vi "Shoot.vi"(5 "Joystick":dbl, 6 "Aimbot?":bool=TRUE, 7 "Aimbot Transformations":T1={"AngleThreshold(degrees)"=100.0, "ShotDuration(10ms)"=100, "PowerScale"=1.0, "AngleShift"=0}, 8 "error in":errorcluster, 9 "Spinup Trigger":bool, 10 "Trigger":bool, 11 "Vision Distance":dbl) -> (0 "error out":errorcluster, 2 "LaunchSpeed(RPM)":dbl, 3 "AngleMotorPosition(Position or %Volts)":dbl)   [LabVIEW 2015]
doc: "Collects and fires boulders according to the following parameters:\n\nTrigger: True will fire the boulder.\nSpinup Trigger: True will spin wheels up prior to firing.\nCollection Trigger: True will spin wheels backwards to collect a boulder.\nAimbot Transformations: Corrective inputs used if we are consistently over/under shooting.\nManual Control: If vision doesn't work, then aim manually using these joystick inputs."
uses:
  Robot Global Data.vi
panel:
  in  "Shot Speed Control":dbl
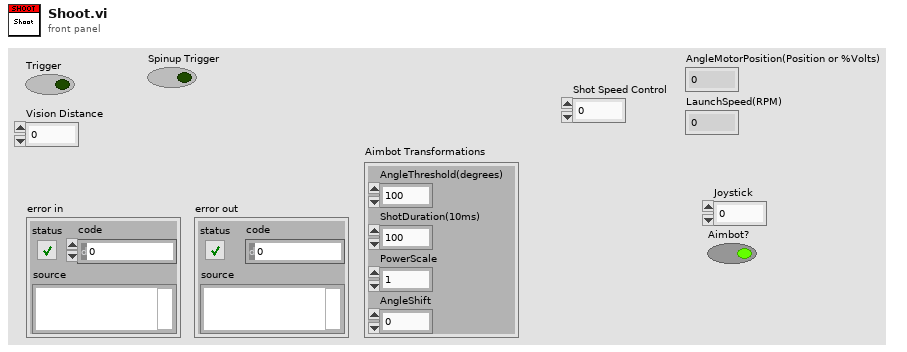
[diagram p1: front panel]
types:
  T1 = cluster{"AngleThreshold(degrees)":dbl, "ShotDuration(10ms)":i32, "PowerScale":dbl, "AngleShift":i32}
  T2 = typedef "Bundle.ctl" = cluster{"error":errorcluster, "AngleMotorRefnum":T3, "LeftWheelRefnum":T3, "RightWheelRefnum":T3, "PushSolenoidRefnum":T10, "AngleMotorPosition(Position or %Volts)":dbl, "LaunchSpeed(RPM)":dbl, "CollectSpeed(RPM)":dbl, "AngleThreshold":dbl, "ShotDuration(10ms)":i32}
  T3 = typedef "WPI_MotorControlDeviceRef.ctl" = cluster{"DeviceStatus":errorcluster, "Type":T4, "PWM":cluster{"PWM Channel":T5, "DeadBand":T6}, "CAN":cluster{"Device Number":u8, "Control Mode":T7, "Semaphore":T8, "Max Vout":dbl, "TalonSRX Control Mode":T9}, "Invert":bool}
  T4 = typedef "WPI_MotorControlType.ctl" = enum16{"PWM", "CAN", "CANTalonSRX"}
  T5 = typedef "FPGA_DIOPWMChannel.ctl" = enum8{"PWM 0", "PWM 1", "PWM 2", "PWM 3", "PWM 4", "PWM 5", "PWM 6", "PWM 7", "PWM 8", "PWM 9", "PWM MXP 0", "PWM MXP 1", "PWM MXP 2", "PWM MXP 3", "PWM MXP 4", "PWM MXP 5", "PWM MXP 6", "PWM MXP 7", "PWM MXP 8", "PWM MXP 9", "Invalid"}
  T6 = typedef "WPI_PWMDeadband.ctl" = cluster{"Name":string, "maxPositivePwm":i32, "minPositivePwm":i32, "centerPwm":i32, "maxNegativePwm":i32, "minNegativePwm":i32, "angularRange":u16}
  T7 = typedef "WPI_CANJaguar_ControlMode.ctl" = enum8{"Percent VBus", "Current", "Speed", "Position", "Voltage"}
  T8 = typedef "Semaphore RefNum" = refnum<k1>
  T9 = typedef "WPI_CANTalonSRX_APIControlMode.ctl" = enum8{"Percent VBus", "Speed", "Position", "Slave", "Unchanged / Invalid", "Voltage Compensation", "Current", "Motion Profile"}
  T10 = typedef "WPI_SolenoidDevRef.ctl" = cluster{"DevStatus":errorcluster, "Pneumatics Control Module":u8, "Forward Solenoid Channel":T11, "Reverse Solenoid Channel":T11}
  T11 = typedef "WPI_SolenoidChannel.ctl" = enum8{"Solenoid 0", "Solenoid 1", "Solenoid 2", "Solenoid 3", "Solenoid 4", "Solenoid 5", "Solenoid 6", "Solenoid 7", "Invalid"}
  T12 = typedef "WPI_DigitalInputDevRef.ctl" = cluster{"DevStatus":errorcluster, "DIO Channel":T13}
  T13 = typedef "FPGA_DIOChannel.ctl" = enum8{"DIO 0", "DIO 1", "DIO 2", "DIO 3", "DIO 4", "DIO 5", "DIO 6", "DIO 7", "DIO 8", "DIO 9", "DIO MXP 0", "DIO MXP 1", "DIO MXP 2", "DIO MXP 3", "DIO MXP 4", "DIO MXP 5", "DIO MXP 6", "DIO MXP 7", "DIO MXP 8", "DIO MXP 9", "DIO MXP 10", "DIO MXP 11", "DIO MXP 12", "DIO MXP 13", "DIO MXP 14", "DIO MXP 15", "Invalid"}
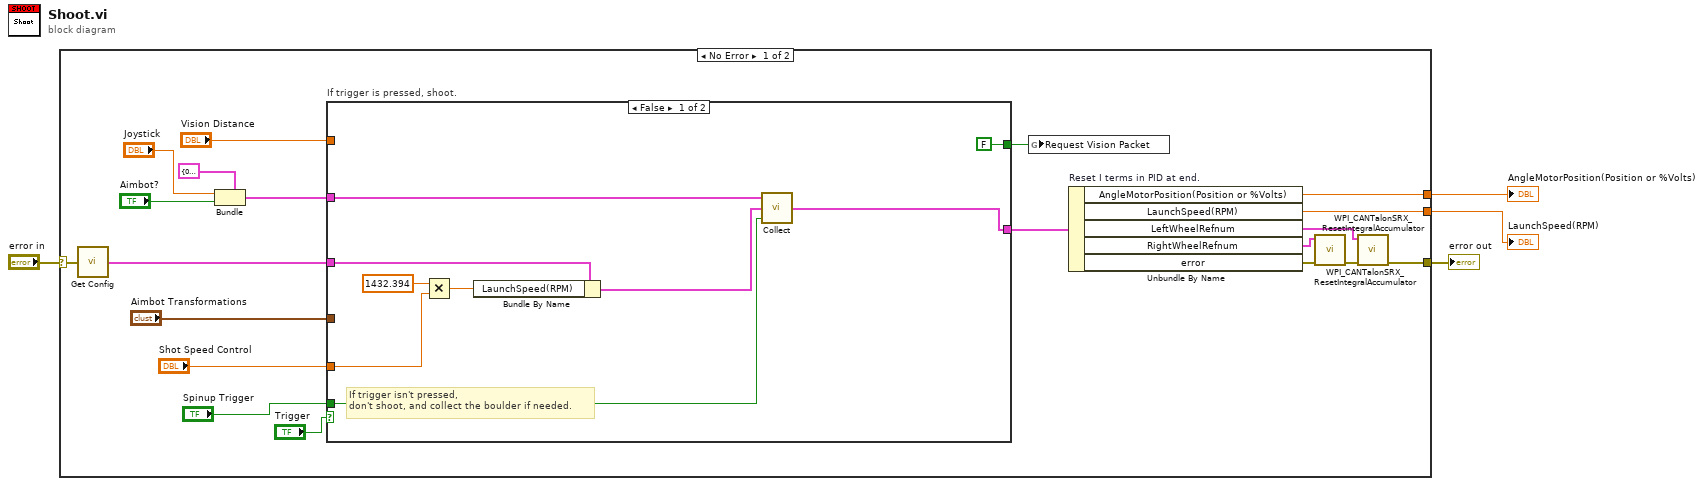
[diagram p0: block diagram]
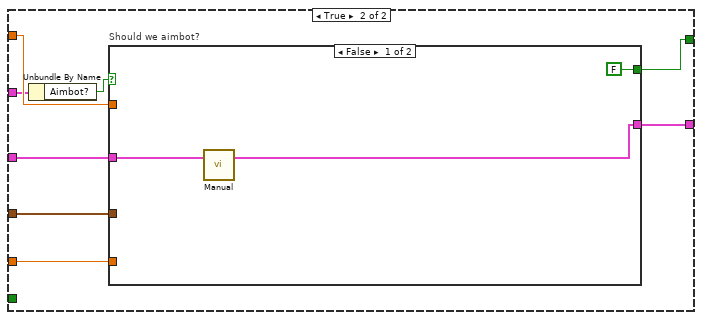
[diagram p2: hidden frame]
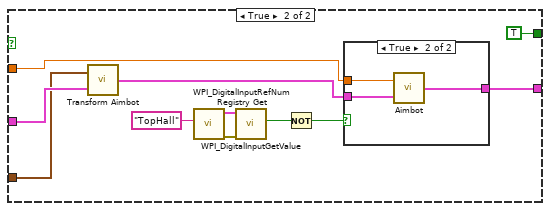
[diagram p3: hidden frame]
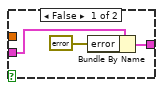
[diagram p4: hidden frame]
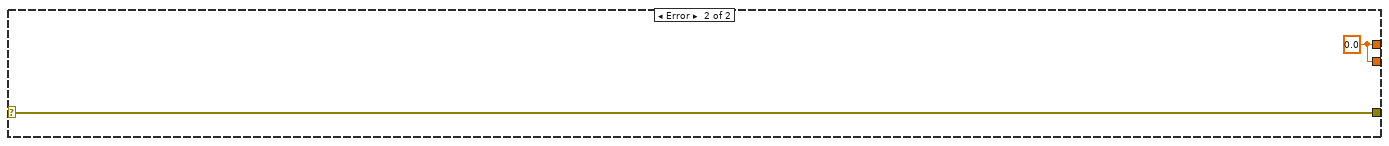
[diagram p5: hidden frame]
diagram:
  n1 = case shown="No Error" "error in" {
    selector: "error in" -> [w14 w63]
    tunnel: [w13 w62] -> w4
    tunnel: [w12 w62] -> w3
    tunnel: [w15 w63] -> w2
    frame No Error {
      n2 = call "Get Config.vi"("error in"=w14) -> ("output cluster"=w6:T2)
      n3 = Bundle(cluster=cluster{"Joystick":dbl, "Aimbot?":bool} {"Joystick"=0.0, "Aimbot?"=TRUE} ("Manual Control"), "Joystick"="Joystick", "Aimbot?"="Aimbot?") -> (w10:cluster{"Joystick":dbl, "Aimbot?":bool})
      n4 = case "If trigger is pressed, shoot." shown="False" "Trigger" {
        tunnel: [w33 w41] -> w22
        tunnel: "Vision Distance" -> [_ w40]
        tunnel: w6 -> [w26 w39]
        tunnel: "Aimbot Transformations" -> [_ w38]
        tunnel: "Spinup Trigger" -> [w32 _]
        tunnel: w10 -> [w31 w37]
        tunnel: [FALSE ("Request Vision Packet") w35] -> w7
        tunnel: "Shot Speed Control" -> [w27 w34]
        frame False {
          # "If trigger isn't pressed,\ndon't shoot, and collect the boulder if needed."
          n5 = Multiply(x=1432.394, y=w27) -> (x*y=w28:dbl)
          n6 = Bundle By Name(cluster=w26, "LaunchSpeed(RPM)"=w28) -> (w25:T2)
          n7 = call "Collect.vi"("SpinupTrigger"=w32, "Firing Data"=w25, "Manual Control"=w31) -> ("Firing Data"=w33:T2)
        }
        frame True {
          n8 = Unbundle By Name(w37) -> ("Aimbot?"=w36:bool)
          n9 = case "Should we aimbot?" shown="False" w36 {
            tunnel: [w44 w47] -> w41
            tunnel: w40 -> [_ w49]
            tunnel: w39 -> [w42 w55]
            tunnel: w38 -> [_ w54]
            tunnel: [FALSE ("Request Vision Packet") TRUE ("Request Vision Packet")] -> w35
            tunnel: w34 -> [_ _]
            frame False {
              n10 = call "Manual.vi"("Firing Data"=w42) -> ("output cluster"=w44:T2)  [unwired: 2 in]
            }
            frame True {
              n11 = call "Transform Aimbot.vi"("Firing Data in"=w55, "Aimbot Transformations"=w54) -> ("Firing Data out"=w48:T2)
              n12 = call <vilib>:"WPI_DigitalInputRefNum Registry Get.vi"("refnum name"="TopHall") -> ("error out"=w45:errorcluster, "DigitalInputDevRef"=w51:T12)  [unwired: 9 in]
              n13 = call <vilib>:"WPI_DigitalInputGetValue.vi"("error in (no error)"=w45, "DigitalInputDevRef"=w51) -> ("Value"=w53:bool)  [unwired: 7 in, 2 out]
              n14 = Not(x=w53) -> (.not. x?=w52:bool)
              n15 = case shown="True" w52 {
                tunnel: w49 -> [_ w61]
                tunnel: w48 -> [w58 w60]
                tunnel: [w56 w59] -> w47
                frame False {
                  n16 = Bundle By Name(cluster=w58, "error"=errorcluster {"status"=TRUE, "code"=9998, "source"="Not at correct angle for shooting!"} ("error constant")) -> (w56:T2)
                }
                frame True {
                  n17 = call "Aimbot.vi"("Firing Data"=w60, "Range"=w61) -> ("Firing Data out"=w59:T2)
                }
              }
            }
          }
        }
      }
      n18 = global write "Robot Global Data.vi" "Request Vision Packet"(w7) -> ()
      n19 = Unbundle By Name "Reset I terms in PID at end."(w22) -> ("AngleMotorPosition(Position or %Volts)"=w12:dbl, "LaunchSpeed(RPM)"=w13:dbl, "LeftWheelRefnum"=w17:T3, "RightWheelRefnum"=w16:T3, "error"=w19:errorcluster)
      n20 = call <vilib>:"WPI_CANTalonSRX_ResetIntegralAccumulator.vi"("error in (no error)"=w19, "CAN Talon SRX Ref"=w16) -> ("error out"=w24:errorcluster)  [unwired: 8 in, 1 out]
      n21 = call <vilib>:"WPI_CANTalonSRX_ResetIntegralAccumulator.vi"("error in (no error)"=w24, "CAN Talon SRX Ref"=w17) -> ("error out"=w15:errorcluster)  [unwired: 8 in, 1 out]
    }
    frame Error {
      w62 = 0.0 ("LaunchSpeed(t/100ms)")
    }
  }
  "error out" <- w2
  "AngleMotorPosition(Position or %Volts)" <- w3
  "LaunchSpeed(RPM)" <- w4
